vi "GL_TempUnits.vi"() -> ()   [LabVIEW 2021]
panel:
  out "unit":enum16{"K", "Ohms", "C", "F"}(ring)
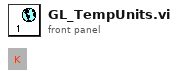
[diagram p1: front panel]
diagram:
